vi "IsTempBackground.vi"(7 "SVG Path":path, 8 "error in":errorcluster, 9 "Order (back to front)":i32, 11 "SVGImage in":refnum<class "SVGImage.lvclass">) -> (0 "error out":errorcluster, 2 "Backgroundic Qualities":T1, 3 "SVGImage out":refnum<class "SVGImage.lvclass">)   [LabVIEW 2019, in "SVGImage.lvclass"]
uses:
  SVGImage.lvclass
  SVGImage.lvclass/SVGImage.ctl
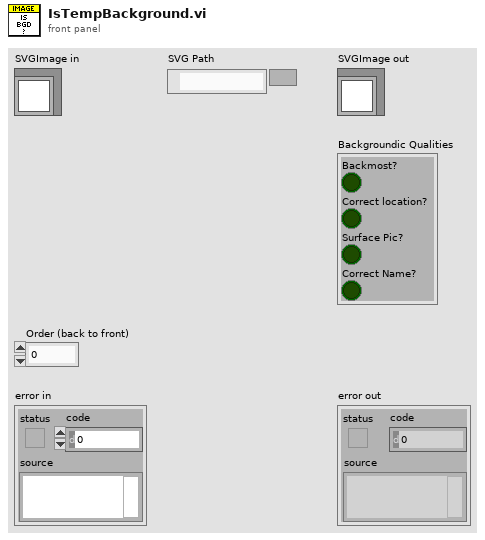
[diagram p1: front panel]
types:
  T1 = cluster{"Backmost?":bool, "Correct location?":bool, "Surface Pic?":bool, "Correct Name?":bool}
  T2 = cluster{"Correct Name?":bool, "Surface Pic?":bool, "Correct location?":bool, "Backmost?":bool}
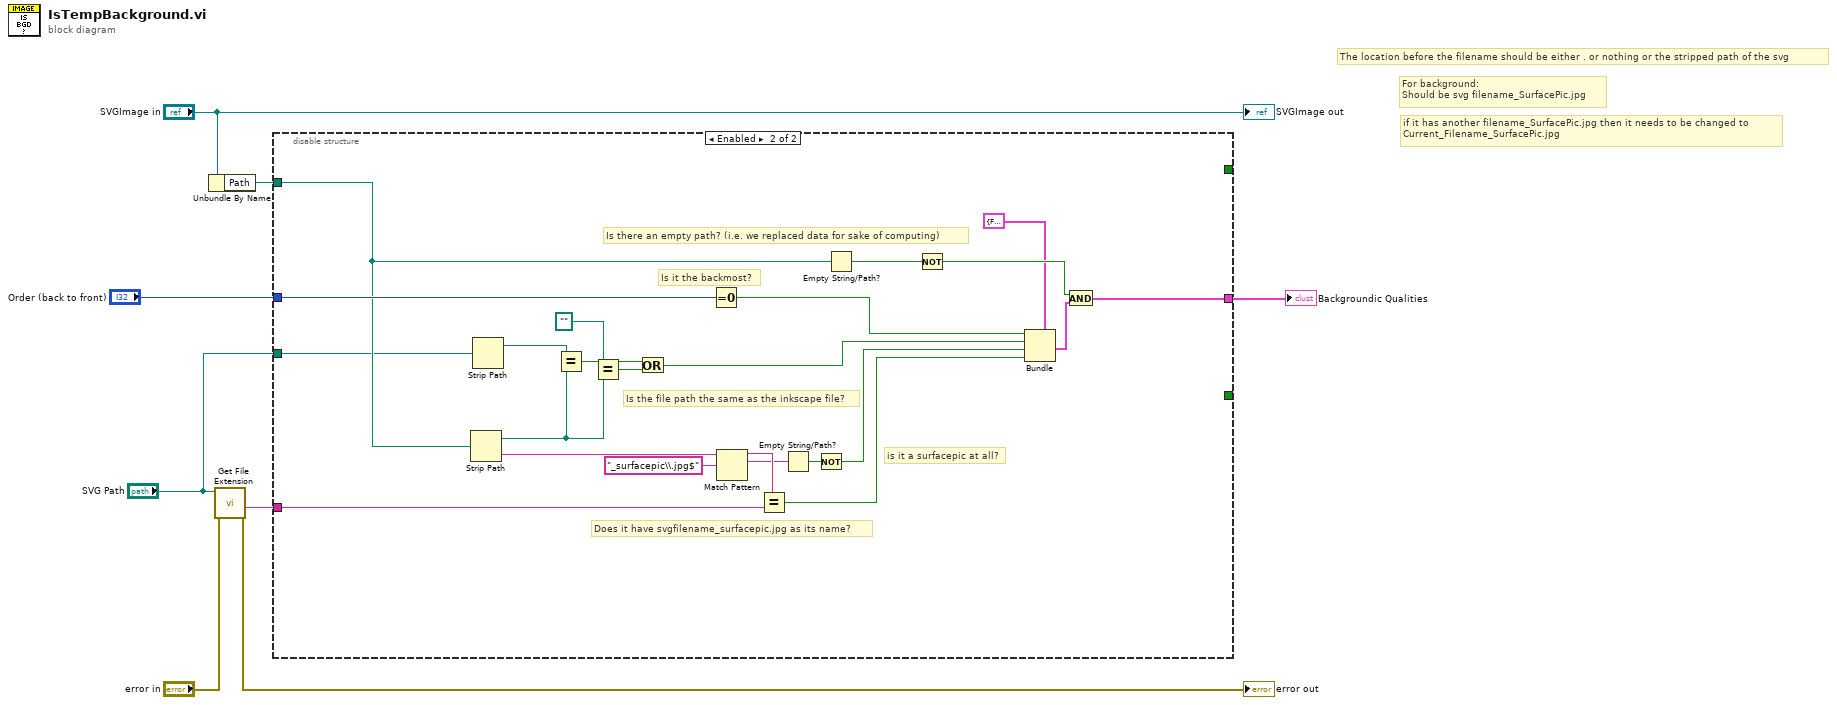
[diagram p0: block diagram]
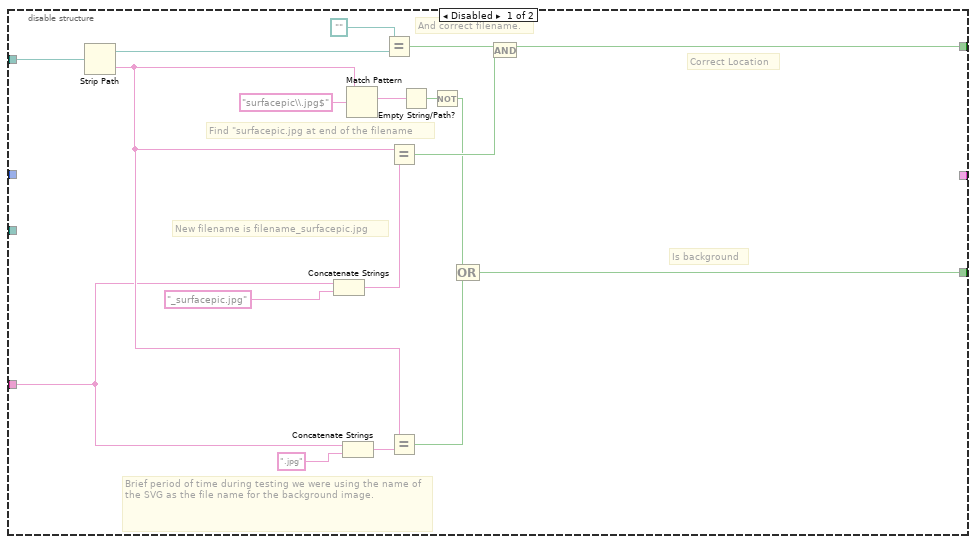
[diagram p2: hidden frame]
diagram:
  # "The location before the filename should be either . or nothing or the stripped path of the svg"
  # "if it has another filename_SurfacePic.jpg then it needs to be changed to \nCurrent_Filename_SurfacePic.jpg"
  # "For background:\nShould be svg filename_SurfacePic.jpg"
  n1 = Unbundle By Name("SVGImage in") -> ("Path"=w6:path)
  n2 = call <vilib>:"Get File Extension.vi"("error in (no error)"="error in", "file"="SVG Path") -> ("error out"=→"error out":errorcluster, "filename without extension"=w4:string)  [unwired: 5 in, 3 out]
  n3 = disable-structure shown="Enabled" {
    disable-tunnel: w6 -> [w22 w33]
    disable-tunnel: [w20 _] -> _
    disable-tunnel: [w16 _] -> _
    disable-tunnel: w4 -> [w9 w32]
    disable-tunnel: "Order (back to front)" -> [_ w34]
    disable-tunnel: [_ w30] -> w2
    disable-tunnel: "SVG Path" -> [_ w29]
    frame Disabled {
      # "Is background"
      # "Correct Location"
      # "New filename is filename_surfacepic.jpg"
      # "Brief period of time during testing we were using the name of the SVG as the file name for the background image."
      # "Find \"surfacepic.jpg at end of the filename"
      # "And correct filename."
      n4 = Strip Path(path=w22) -> (stripped path=w25:path, name=w10:string)
      n5 = Concatenate Strings(w9, "_surfacepic.jpg" ("string")) -> (w17:string)
      n6 = Concatenate Strings(w9, ".jpg" ("string")) -> (w12:string)
      n7 = Match Pattern(string=w10, regular expression="surfacepic\\.jpg$") -> (match substring=w23:string)  [unwired: 1 in, 3 out]
      n8 = Equal?(x=path "", y=w25) -> (x = y?=w19:bool)
      n9 = Equal?(x=w10, y=w17) -> (x = y?=w15:bool)
      n10 = Equal?(x=w10, y=w12) -> (x = y?=w11:bool)
      n11 = Empty String/Path?(string/path=w23) -> (empty?=w21:bool)
      n12 = Not(x=w21) -> (.not. x?=w14:bool)
      n13 = Compound Arithmetic op=OR(w14, w11) -> (w20:bool)
      n14 = And(x=w19, y=w15) -> (x .and. y?=w16:bool)
    }
    frame Enabled {
      # "Is there an empty path? (i.e. we replaced data for sake of computing)"
      # "Is it the backmost?"
      # "Is the file path the same as the inkscape file?"
      # "is it a surfacepic at all?"
      # "Does it have svgfilename_surfacepic.jpg as its name?"
      n15 = Strip Path(path=w33) -> (stripped path=w28:path, name=w38:string)
      n16 = Strip Path(path=w29) -> (stripped path=w27:path)  [unwired: 1 out]
      n17 = Equal?(x=w27, y=w28) -> (x = y?=w43:bool)
      n18 = Equal?(x=path "", y=w28) -> (x = y?=w44:bool)
      n19 = Or(x=w43, y=w44) -> (x .or. y?=w40:bool)
      n20 = Equal To 0?(x=w34) -> (x = 0?=w39:bool)
      n21 = Match Pattern(string=w38, regular expression="_surfacepic\\.jpg$") -> (before substring=w48:string, match substring=w47:string)  [unwired: 1 in, 2 out]
      n22 = Equal?(x=w48, y=w32) -> (x = y?=w42:bool)
      n23 = Empty String/Path?(string/path=w47) -> (empty?=w46:bool)
      n24 = Not(x=w46) -> (.not. x?=w41:bool)
      n25 = Empty String/Path?(string/path=w33) -> (empty?=w37:bool)
      n26 = Not(x=w37) -> (.not. x?=w36:bool)
      n27 = Bundle(cluster=T2 {"Correct Name?"=FALSE, "Surface Pic?"=FALSE, "Correct location?"=FALSE, "Backmost?"=FALSE}, "Correct Name?"=w39, "Surface Pic?"=w40, "Correct location?"=w41, "Backmost?"=w42) -> (w35:T2)
      n28 = And(x=w36, y=w35) -> (x .and. y?=w30:T2)
    }
  }
  "Backgroundic Qualities" <- w2
  "SVGImage out" <- "SVGImage in"
